vi "Set Initialization Data - DAQ Worker.vi"(8 "error in":errorcluster, 11 "ChartView in":refnum<class "ChartView.lvclass">) -> (0 "error out":errorcluster, 3 "ChartView out":refnum<class "ChartView.lvclass">)   [LabVIEW 2020, in "ChartView.lvclass"]
doc: "In this VI you can set the initialization data of a statically-linked subWorker."
uses:
  ChartView.lvclass
  DAQ Worker/Initialization Data.ctl
  DAQ Worker/Response Cases.ctl
  ChartView.lvclass/ChartView.ctl
  DAQ Worker/DAQ Worker.lvclass
  C:/Program Files (x86)/National Instruments/LabVIEW 2020/vi.lib/addons/_Workers/Library/Classes/Worker/Worker.lvclass
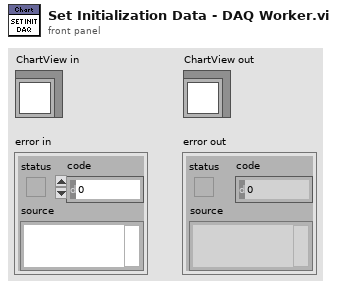
[diagram p1: front panel]
types:
  T1 = typedef "DAQ Worker.lvclass/Initialization Data.ctl" = cluster{"Response Cases":T2}
  T2 = typedef "DAQ Worker.lvclass/Response Cases.ctl" = cluster{"Placeholder - Can be deleted":string}
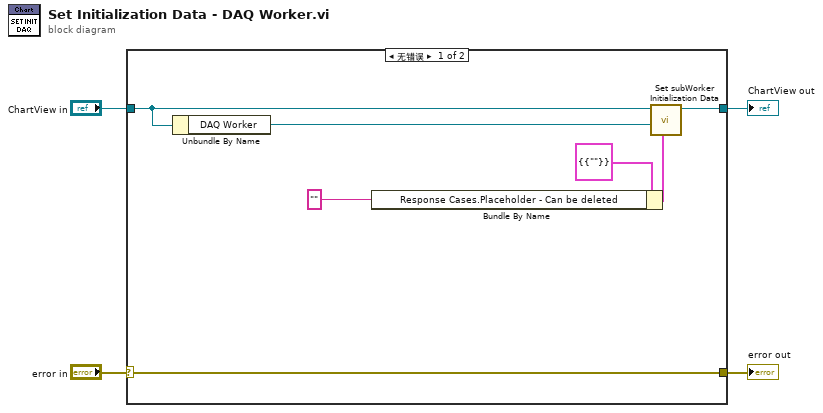
[diagram p0: block diagram]
diagram:
  n1 = case shown="无错误" "error in" {
    selector: "error in" -> [w11 w13]
    tunnel: [w11 w13] -> w3
    tunnel: [w9 w12] -> w2
    tunnel: "ChartView in" -> [w8 w12]
    frame No Error {
      n2 = Unbundle By Name(w8) -> ("DAQ Worker"=w10:refnum<class "DAQ Worker.lvclass">)
      n3 = Bundle By Name(cluster=T1 {"Response Cases"={"Placeholder - Can be deleted"=""}} ("Initialization Data"), "Response Cases.Placeholder - Can be deleted"="" ("Placeholder")) -> (w6:T1)
      n4 = call-dynamic "Set subWorker Initialization Data.vi"("Initialization Data"=w6, "subWorker"=w10, "Worker"=w8) -> ("Worker out"=w9:refnum<class "ChartView.lvclass">)  [unwired: 8 in]
    }
    frame Error {
    }
  }
  "error out" <- w3
  "ChartView out" <- w2
